vi "Get Alarm State.vi"(11 "error in (no error)":errorcluster) -> (8 "Alarm state":string[][](array[string]), 14 "updated":bool, 15 "error out":errorcluster)   [LabVIEW 2011]
uses:
  E&S/Monitor/Actino S&E monitor.ctl
  Measurments Handling/Action Analog Handler.ctl
  E&S/String outpyt type.ctl
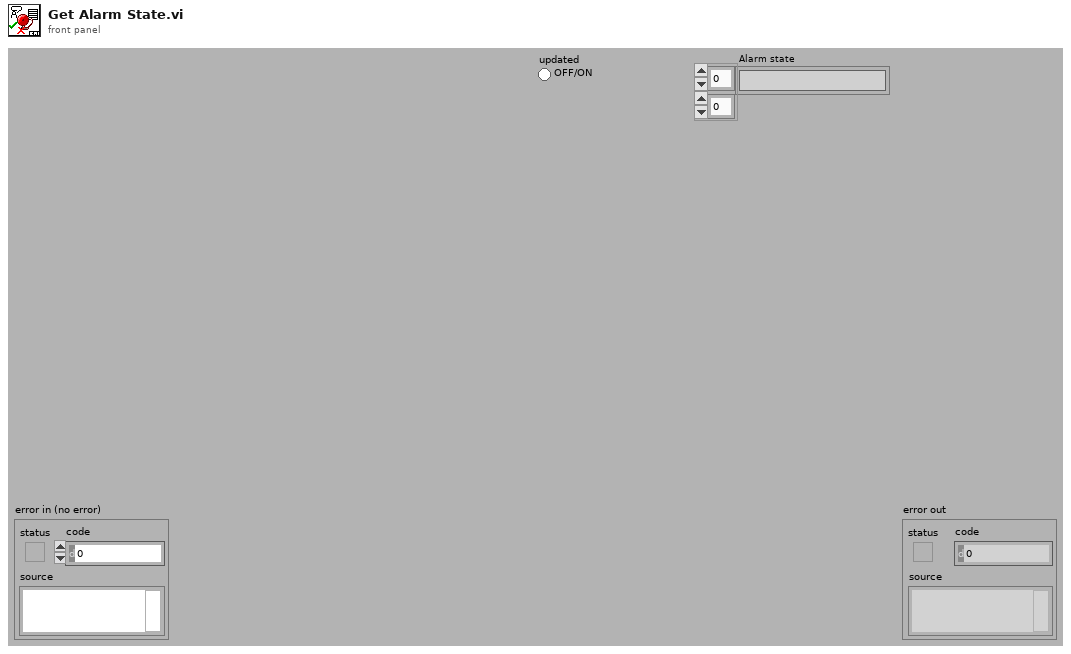
[diagram p1: front panel]
types:
  T1 = typedef "Actino S&E monitor.ctl" = enum16{"GET(type history)", "SET S&E", "(Re)Init", "Get Error state", "Get  Alarm state", "Get All", "Get last  250", "Get Alarm History"}
  T2 = typedef "_emi_ S&E Message.ctl" = cluster{"Type":T3, "Originate time":dbl, "System":u8, "Loop":u16, "Sub ID":u16, "Elevated priority":bool, "E&S Message content":variant}
  T3 = typedef "_emi_ S&E Message type.ctl" = enum16{"Error/Warning", "Note", "Debug", "Event", "Alarm Analog", "Alarm Digital", "Annotation"}
  T4 = typedef "String outpyt type.ctl" = enum16{"Full File hist", "Simple File hist", "Displ Hist one type", "Displ Hist mult types", "Displ Stat one type", "Displ Stat Mult type"}
  T5 = typedef "Action Analog Handler.ctl" = enum16{"GET value", "GET Single Frequenzy", "GET All Values", "GET Waveform", "Get Numb Var", "SET Value", "START Buffer", "REG Variable", "BUF size(total antal sekund)", "PULS", "Get a Value at time", "Set initial waveform"}
  T6 = typedef "Status Digitalish.ctl" = enum16{"NA", "False", "True"}
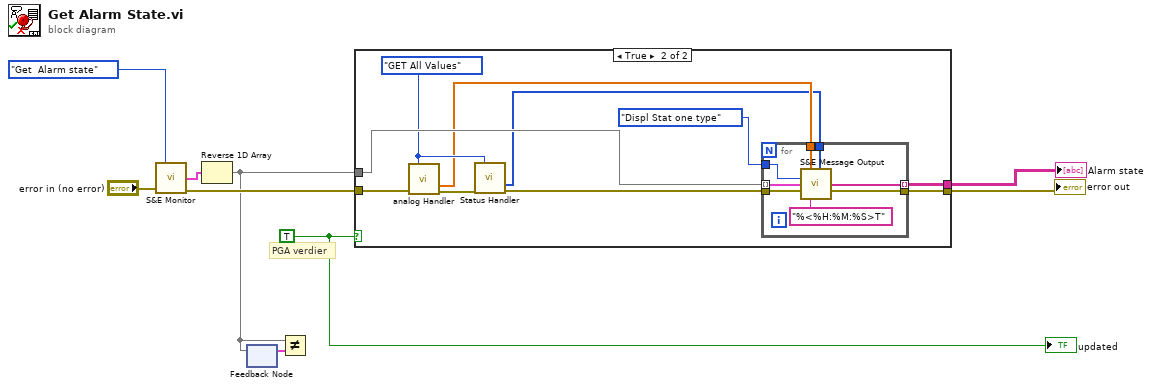
[diagram p0: block diagram]
diagram:
  w1 = TRUE
  # "PGA verdier"
  n1 = call "S&E Monitor.vi"("Action(GET 250)"=Actino_S&E_monitor."Get  Alarm state", "error in (no error)"="error in (no error)") -> ("S&E"=w7:T2[], "error out"=w5:errorcluster)  [unwired: 12 in]
  n2 = Reverse 1D Array(array=w7) -> (reversed array=w4:T2[])
  n3 = feedback-in #1(w4) -> ()
  n4 = feedback #1() -> (w6:T2[])  [unwired: 1 in]
  n5 = Not Equal?(x=w4, y=w6) -> ()  [unwired: 1 out]
  n6 = case shown="True" w1 {
    tunnel: w5 -> [w10 w16]
    tunnel: w4 -> [_ w17]
    tunnel: [w10 w19] -> w2
    tunnel: [_ w18] -> w3
    frame False {
    }
    frame True {
      w13 = Action_Analog_Handler."GET All Values" ("Action")
      n7 = call "analog Handler.vi"("Action"=w13, "error in (no error)"=w16) -> ("Values"=w12:dbl[], "error out"=w15:errorcluster)  [unwired: 8 in, 4 out]
      n8 = call "Status Handler.vi"("Action"=w13, "error in (no error)"=w15) -> ("Values"=w11:T6[], "error out"=w14:errorcluster)  [unwired: 9 in, 3 out]
      n9 = for {
        tunnel: String_outpyt_type."Displ Stat one type" ("Type(File Hist)") -> [w28]
        tunnel: w14 -> [w27]
        tunnel: w17 -> [w26] mode=indexing
        tunnel: [w25] -> w19
        tunnel: [w23] -> w18 mode=indexing
        tunnel: w12 -> [w22]
        tunnel: w11 -> [w21]
        n10 = call "S&E Message Output.vi"("All analog ch data"=w22, "All digital Ch data"=w21, "Type(File Hist)"=w28, "E&S Message"=w26, "error in (no error)"=w27, "Time format(%T)"="%<%H:%M:%S>T") -> ("Array of strings"=w23:string[], "error out"=w25:errorcluster)  [unwired: 7 in, 1 out]
      }
    }
  }
  "error out" <- w2
  "Alarm state" <- w3
  "updated" <- w1
